vi "Connect.vi"(8 "error in":errorcluster, 11 "Kronos in":refnum<class "Kronos.lvclass">) -> (0 "error out":errorcluster, 3 "Kronos out":refnum<class "Kronos.lvclass">)   [LabVIEW 2018, in "Kronos.lvlib" / "Kronos.lvclass"]
uses:
  Kronos.lvclass
  Custom Controls/Serial Settings.ctl
  PPLs/Laser/Parent/Laser.lvlibp/Custom Controls/Command List.ctl
  <vilib>/Instr/_visa.llb/VISA Configure Serial Port (Instr).vi
  PPLs/Laser/Parent/Laser.lvlibp/Laser.lvclass
  Kronos.lvlib
  C:/AME Test Engineering/LabVIEW/PPLs/Laser/Parent/Laser.lvlibp/Laser.lvclass
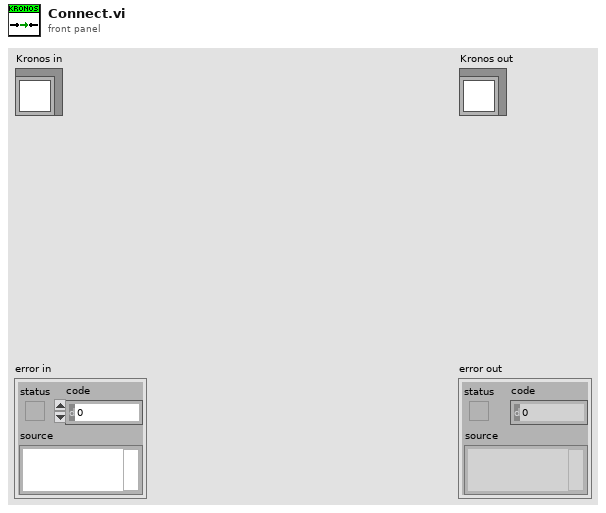
[diagram p1: front panel]
types:
  T1 = typedef "Laser.lvlibp/Laser.lvclass/Command List.ctl" = enum16{"None", "Config?", "Volt?", "ThCase?", "STS?", "Mon?", "Help?", "HB", "Verbose", "Spnt", "Ext", "PRF", "Start", "Stop", "PRF?", "State?", "Status?", "Stat?", "Read HB", "Logon", "Poutmax", "saveconfig", "Reset", "Poutmax?", "PoutCommandMax", "PoutCommandMax?", "FreqMin", "FreqMin?"}
  T2 = typedef "Kronos.lvlib/Serial Settings.ctl" = cluster{"Enable Termination\nChar (T)":bool, "termination char\n(0xA = '\\n' = LF) ":u8, "timeout (10sec)":u32, "baud rate (9600)":u32, "data bits (8)":u16, "parity (0:none)":enum16{"None", "Odd", "Even", "Mark", "Space"}, "stop bits (10: 1 bit)":u16, "flow control (0:none)":enum16{"None", "XON/XOFF", "RTS/CTS", "XON/XOFF & RTS/CTS", "DTR/DSR", "XON/XOFF & DTR/DSR"}}
  T3 = enum16{"None", "XON/XOFF", "RTS/CTS", "XON/XOFF & RTS/CTS", "DTR/DSR", "XON/XOFF & DTR/DSR"}
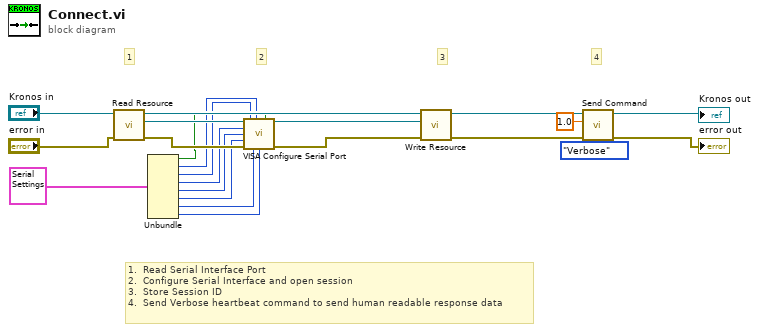
[diagram p0: block diagram]
diagram:
  # "1.  Read Serial Interface Port\n2.  Configure Serial Interface and open session\n3.  Store Session ID\n4.  Send Verbose heartbeat command to send human readable response data"
  # "4"
  # "3"
  # "2"
  # "1"
  n1 = call "Read Resource.vi"("error in (no error)"="error in", "Laser in"="Kronos in") -> ("error out"=w19:errorcluster, "Resource"=w17:refnum<visa-resource-name>, "Laser out"=w21:refnum<class "Kronos.lvclass">)  [unwired: 7 in]
  n2 = Unbundle(T2 {"Enable Termination\nChar (T)"=FALSE, "termination char\n(0xA = '\\n' = LF) "=10, "timeout (10sec)"=100, "baud rate (9600)"=19200, "data bits (8)"=8, "parity (0:none)"=enum."None", "stop bits (10: 1 bit)"=10, "flow control (0:none)"=enum."None"} ("Serial Settings")) -> ("Enable Termination\nChar (T)"=w14:bool, "termination char\n(0xA = '\\n' = LF)"=w13:u8, "timeout (10sec)"=w12:u32, "baud rate (9600)"=w11:u32, "data bits (8)"=w10:u16, "parity (0:none)"=w9:enum16{"None", "Odd", "Even", "Mark", "Space"}, "stop bits (10: 1 bit)"=w8:u16, "flow control (0:none)"=w7:T3)
  n3 = call-poly "VISA Configure Serial Port"("VISA resource name"=w17, "timeout (10sec)"=w12, "termination char\n(0xA = '\\n' = LF)"=w13, "Enable Termination\nChar (T)"=w14, "baud rate (9600)"=w11, "data bits (8)"=w10, "parity (0:none)"=w9, "error in (no error)"=w19, "stop bits (10: 1 bit)"=w8, "flow control (0:none)"=w7) -> ("VISA resource name out"=w16:refnum<visa-resource-name>, "error out"=w18:errorcluster)  [unwired: 4 in]
  n4 = call "Write Resource.vi"("error in (no error)"=w18, "Resource"=w16, "Laser in"=w21) -> ("error out"=w2:errorcluster, "Laser out"=w6:refnum<class "Kronos.lvclass">)  [unwired: 7 in]
  n5 = call-dynamic "Send Command.vi"("Command in"=Command_List."Verbose" ("Command"), "error in"=w2, "Value"=1.0, "Kronos in"=w6) -> ("error out"=→"error out":errorcluster, "Kronos out"=→"Kronos out":refnum<class "Kronos.lvclass">)  [unwired: 5 in, 1 out]
